vi "debugger Index Files.vi"(7 "ENV":T1, 8 "error in (no error)":errorcluster, 10 "Serial Number":string, 11 "Model Number":string) -> (0 "error out":errorcluster, 1 "Template Keys":T1)   [LabVIEW 2011]
uses:
  ITK EXT/utils/keyedarr.llb/Keyed Array.ctl
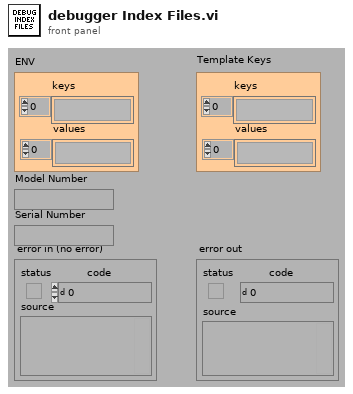
[diagram p1: front panel]
types:
  T1 = typedef "Keyed Array.ctl" = cluster{"keys":string[], "values":string[]}
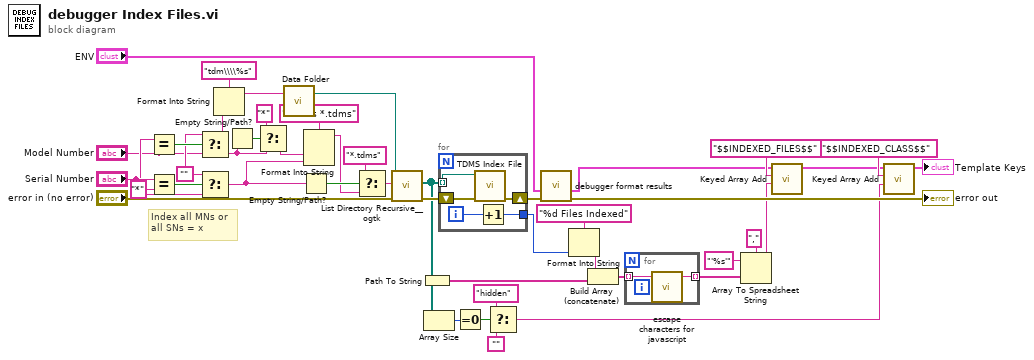
[diagram p0: block diagram]
diagram:
  w29 = ""
  w31 = "*" ("y")
  # "Index all MNs or\nall SNs = x"
  n1 = Equal?(x=w31, y="Model Number") -> (x = y?=w30:bool)
  n2 = Equal?(x="Serial Number", y=w31) -> (x = y?=w34:bool)
  n3 = Select(t=w29, s=w30, f="Model Number") -> (s? t:f=w28:string)
  n4 = Select(t=w29, s=w34, f="Serial Number") -> (s? t:f=w32:string)
  n5 = Format Into String(format string="tdm\\\\%s", w28) -> (resulting string=w43:string)  [unwired: 2 in, 1 out]
  n6 = Empty String/Path?(string/path="Model Number") -> (empty?=w14:bool)
  n7 = Select(t="*" ("y"), s=w14, f="Model Number") -> (s? t:f=w12:string)
  n8 = call "Data Folder.vi"("Relative Path (\"\" - Folder)"=w43) -> ("Data Folder"=w36:path)  [unwired: 2 in]
  n9 = Empty String/Path?(string/path=w32) -> (empty?=w40:bool)
  n10 = Format Into String(format string="%s %s *.tdms" ("pattern"), w12, w32) -> (resulting string=w38:string)  [unwired: 2 in, 1 out]
  n11 = Select(t="*.tdms" ("pattern"), s=w40, f=w38) -> (s? t:f=w37:string)
  n12 = call "List Directory Recursive__ogtk.vi"("error in (no error)"="error in (no error)", "pattern"=w37, "Path"=w36) -> ("error out"=w42:errorcluster, "file paths"=w7:path[])  [unwired: 5 in, 2 out]
  n13 = Path To String(path=w7) -> (string=w16:string[])
  n14 = Array Size(array=w7) -> (size(s)=w6:i32)
  n15 = for {
    shift-right: [w48] -> w27
    shift-left: w42 -> [w49]
    tunnel: w7 -> [w47] mode=indexing
    tunnel: [w45] -> w1
    i -> [w46]
    n16 = call "TDMS Index File.vi"("error in (no error)"=w49, "TDMS File Path"=w47) -> ("error out"=w48:errorcluster)  [unwired: 8 in, 1 out]
    n17 = Increment(x=w46) -> (x+1=w45:i32)
  }
  n18 = Equal To 0?(x=w6) -> (x = 0?=w5:bool)
  n19 = Select(t="hidden" ("key"), s=w5, f="") -> (s? t:f=w2:string)
  n20 = call "debugger format results.vi"("error in (no error)"=w27, "ENV"="ENV") -> ("error out"=→"error out":errorcluster, "Template Keys"=w23:T1)  [unwired: 3 in, 5 out]
  n21 = Format Into String(format string="%d Files Indexed", w1) -> (resulting string=w17:string)  [unwired: 2 in, 1 out]
  n22 = Build Array (concatenate)(w17, w16) -> (w15:string[])
  n23 = for {
    tunnel: w15 -> [w50] mode=indexing
    tunnel: [w51] -> w21 mode=indexing
    n24 = call "escape characters for javascript.vi"("String (\"\")"=w50) -> ("escaped String"=w51:string)  [unwired: 4 out]
  }
  n25 = Array To Spreadsheet String(delimiter (Tab)="," ("key"), array=w21, 3:"'%s'" ("key")) -> (spreadsheet string=w18:string)
  n26 = call "Keyed Array Add.vi"("value"=w18, "key"="$$INDEXED_FILES$$", "array in"=w23) -> ("array out"=w9:T1)  [unwired: 2 in, 2 out]
  n27 = call "Keyed Array Add.vi"("value"=w2, "key"="$$INDEXED_CLASS$$", "array in"=w9) -> ("array out"=→"Template Keys":T1)  [unwired: 2 in, 2 out]
